vi "Config_Change.vi"(8 "error in (no error)":errorcluster, 9 "Simulated Signal ?":bool, 11 "Config In":T2) -> (0 "error out":errorcluster, 3 "Config Out":T2)   [LabVIEW 2024]
uses:
  controls/Config_Settings.ctl
panel:
  in  "Square Wave Duty Cycle":dbl format="%#_g%"
  in  "Number of Samples":dbl
  in  "Samples per Sec":dbl
  in  "Cancel":bool
  in  "OK":bool
  in  "signal type":T1(ring)
  in  "Noise Amplitude":dbl
  in  "Offset":dbl
  in  "Phase":dbl
  in  "Frequency":dbl
  in  "Amplitude":dbl
  # "Samples \nper Second"
  # "Number of \nSamples"
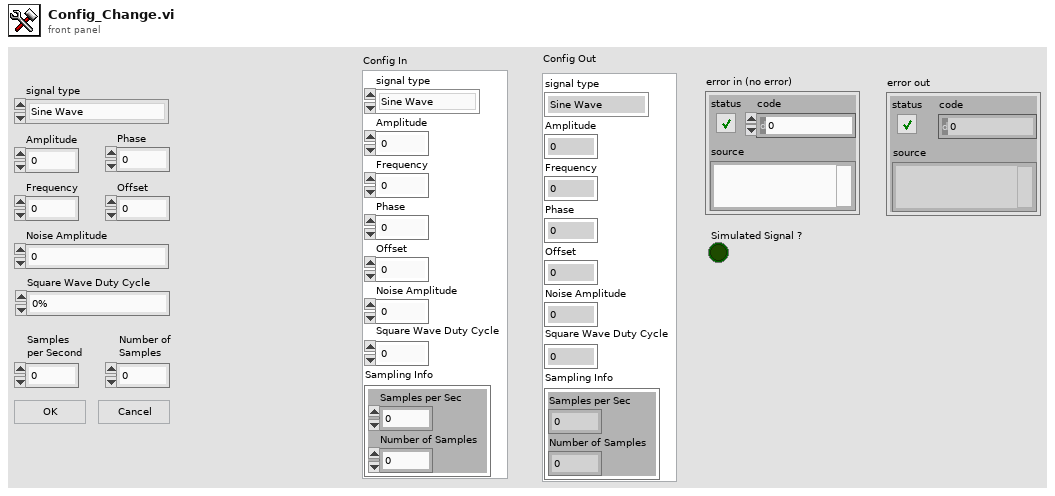
[diagram p1: front panel]
types:
  T1 = enum16{"Sine Wave", "Triangle Wave", "Square Wave", "Sawtooth Wave"}
  T2 = typedef "Config_Settings.ctl" = cluster{"signal type":enum16{"Sine Wave", "Triangle Wave", "Square Wave", "Sawtooth Wave"}, "Amplitude":dbl, "Frequency":dbl, "Phase":dbl, "Offset":dbl, "Noise Amplitude":dbl, "Square Wave Duty Cycle":dbl, "Sampling Info":cluster{"Samples per Sec":dbl, "Number of Samples":dbl}}
  T3 = enum8{"Enabled", "Disabled", "Disabled and Grayed Out"}
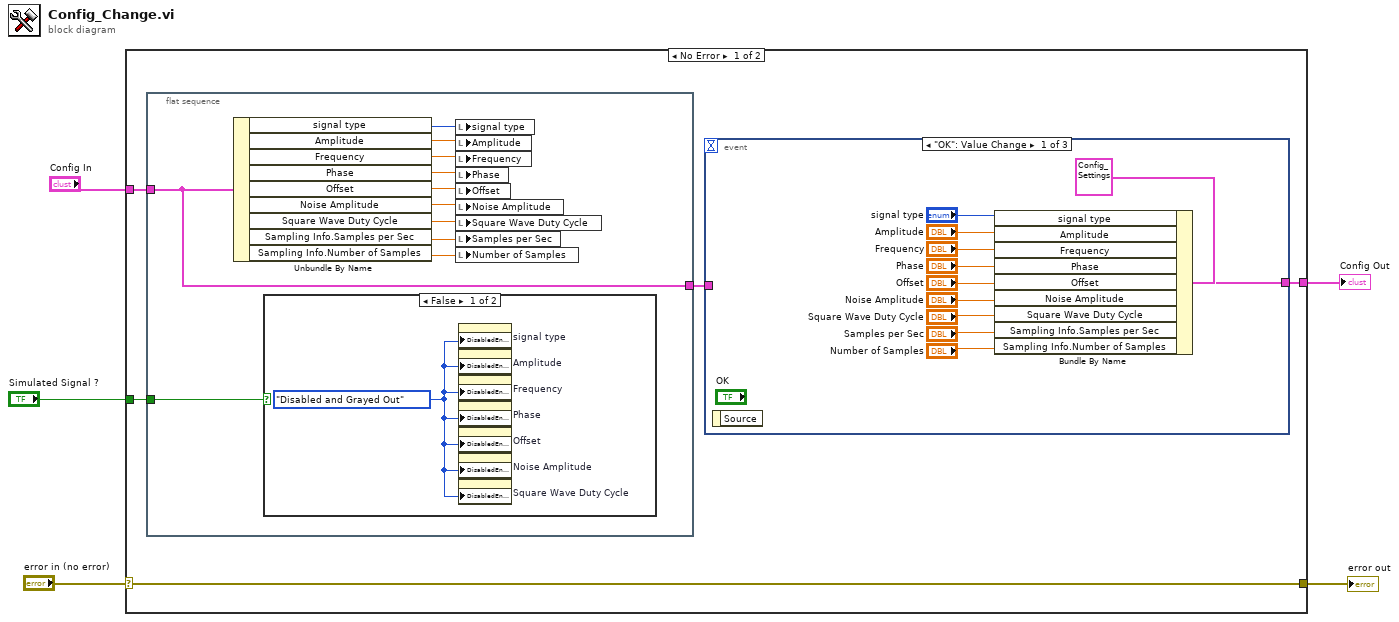
[diagram p0: block diagram]
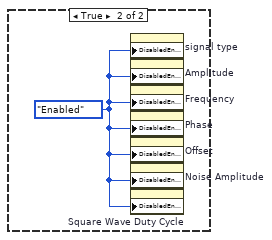
[diagram p2: hidden frame]
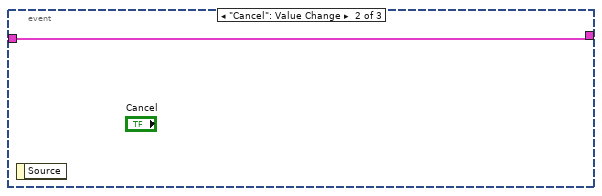
[diagram p3: hidden frame]
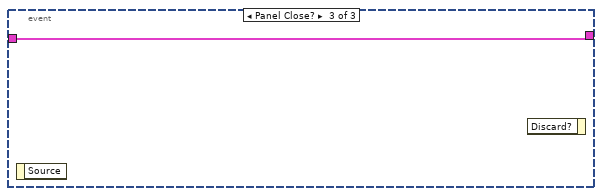
[diagram p4: hidden frame]
diagram:
  n1 = case shown="No Error" "error in (no error)" {
    selector: "error in (no error)" -> [w10 w37]
    tunnel: [w10 w37] -> w4
    tunnel: "Config In" -> [w9 w38]
    tunnel: [w7 w38] -> w2
    tunnel: "Simulated Signal ?" -> [w6 _]
    frame No Error {
      n2 = flat-sequence {
        tunnel: w9 -> [w15]
        tunnel: [w15] -> w8
        tunnel: w6 -> [w12]
        frame #0 {
          n3 = Unbundle By Name(w15) -> ("signal type"=w21:T1, "Amplitude"=w16:dbl, "Frequency"=w17:dbl, "Phase"=w18:dbl, "Offset"=w19:dbl, "Noise Amplitude"=w20:dbl, "Square Wave Duty Cycle"=w11:dbl, "Sampling Info.Samples per Sec"=w14:dbl, "Sampling Info.Number of Samples"=w13:dbl)
          n4 = case shown="False" w12 {
            frame False {
              w22 = T3."Disabled and Grayed Out" ("Disabled")
              n5 = property on="signal type" class="Enum (strict)"("DisabledEnum"=w22) -> ()  [unwired: 2 in, 2 out]
              n6 = property on="Amplitude" class="DigNum (strict)"("DisabledEnum"=w22) -> ()  [unwired: 2 in, 2 out]
              n7 = property on="Frequency" class="DigNum (strict)"("DisabledEnum"=w22) -> ()  [unwired: 2 in, 2 out]
              n8 = property on="Phase" class="DigNum (strict)"("DisabledEnum"=w22) -> ()  [unwired: 2 in, 2 out]
              n9 = property on="Offset" class="DigNum (strict)"("DisabledEnum"=w22) -> ()  [unwired: 2 in, 2 out]
              n10 = property on="Noise Amplitude" class="DigNum (strict)"("DisabledEnum"=w22) -> ()  [unwired: 2 in, 2 out]
              n11 = property on="Square Wave Duty Cycle" class="DigNum (strict)"("DisabledEnum"=w22) -> ()  [unwired: 2 in, 2 out]
            }
            frame True {
              w23 = T3."Enabled" ("Disabled")
              n12 = property on="signal type" class="Enum (strict)"("DisabledEnum"=w23) -> ()  [unwired: 2 in, 2 out]
              n13 = property on="Amplitude" class="DigNum (strict)"("DisabledEnum"=w23) -> ()  [unwired: 2 in, 2 out]
              n14 = property on="Frequency" class="DigNum (strict)"("DisabledEnum"=w23) -> ()  [unwired: 2 in, 2 out]
              n15 = property on="Phase" class="DigNum (strict)"("DisabledEnum"=w23) -> ()  [unwired: 2 in, 2 out]
              n16 = property on="Offset" class="DigNum (strict)"("DisabledEnum"=w23) -> ()  [unwired: 2 in, 2 out]
              n17 = property on="Noise Amplitude" class="DigNum (strict)"("DisabledEnum"=w23) -> ()  [unwired: 2 in, 2 out]
              n18 = property on="Square Wave Duty Cycle" class="DigNum (strict)"("DisabledEnum"=w23) -> ()  [unwired: 2 in, 2 out]
            }
          }
          n19 = local write "signal type"(w21) -> ()
          n20 = local write "Amplitude"(w16) -> ()
          n21 = local write "Frequency"(w17) -> ()
          n22 = local write "Phase"(w18) -> ()
          n23 = local write "Offset"(w19) -> ()
          n24 = local write "Noise Amplitude"(w20) -> ()
          n25 = local write "Square Wave Duty Cycle"(w11) -> ()
          n26 = local write "Samples per Sec"(w14) -> ()
          n27 = local write "Number of Samples"(w13) -> ()
        }
      }
      n28 = event shown="[0] \"OK\": Value Change" {
        selector: _ -> [_ _ _]
        dyn-events: _ -> [_ _ _]
        timeout: _ -> [_ _ _]
        tunnel: w8 -> [_ w35 w36]
        tunnel: [w27 w35 w36] -> w7
        event "OK": Value Change {
          n29 = event-data() -> ()  [unwired: 1 in, 1 out]
          n30 = Bundle By Name(cluster=T2 {"signal type"=enum."Sawtooth Wave", "Amplitude"=0.0, "Frequency"=0.0, "Phase"=0.0, "Offset"=0.0, "Noise Amplitude"=0.0, "Square Wave Duty Cycle"=0.0, "Sampling Info"={"Samples per Sec"=0.0, "Number of Samples"=0.0}} ("Config Settings"), "signal type"="signal type", "Amplitude"="Amplitude", "Frequency"="Frequency", "Phase"="Phase", "Offset"="Offset", "Noise Amplitude"="Noise Amplitude", "Square Wave Duty Cycle"="Square Wave Duty Cycle", "Sampling Info.Samples per Sec"="Samples per Sec", "Sampling Info.Number of Samples"="Number of Samples") -> (w27:T2)
        }
        event "Cancel": Value Change {
          n31 = event-data() -> ()  [unwired: 1 in, 1 out]
        }
        event Panel Close? {
          n32 = event-data() -> ()  [unwired: 1 in, 1 out]
          n33 = event-data() -> ()  [unwired: 2 in, 1 out]
        }
      }
    }
    frame Error {
    }
  }
  "Config Out" <- w2
  "error out" <- w4
